vi "Heapify.vi"(8 "error in (no error)":errorcluster, 10 "index":i32, 11 "Astar Open List in":refnum<class "NI_Robotics_Priority Queue.lvclass">) -> (0 "error out":errorcluster, 3 "Astar Open List out":refnum<class "NI_Robotics_Priority Queue.lvclass">)   [LabVIEW 2017, in "NI_Robotics_Priority Queue.lvclass"]
uses:
  <vilib>/robotics/Navigation/shared/Priority Queue/NI_Robotics_Priority Queue.lvclass
panel:
  in  "up heap (F)":bool
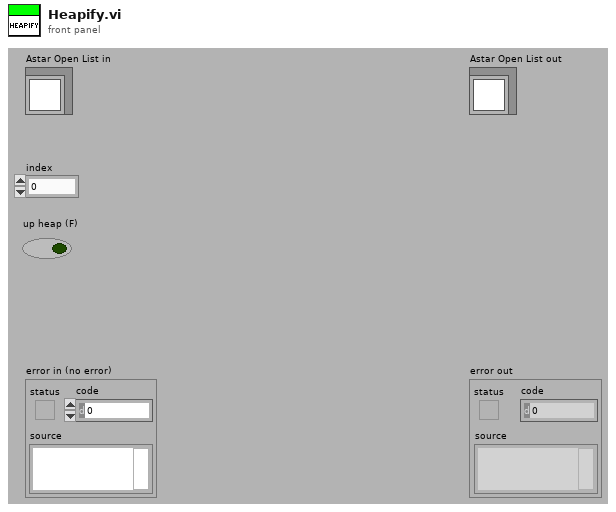
[diagram p1: front panel]
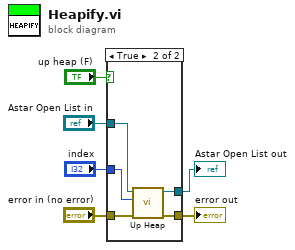
[diagram p0: block diagram]
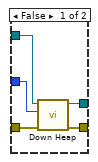
[diagram p2: hidden frame]
diagram:
  n1 = case shown="True" "up heap (F)" {
    tunnel: "Astar Open List in" -> [w11 w16]
    tunnel: "index" -> [w10 w15]
    tunnel: [w9 w13] -> w3
    tunnel: "error in (no error)" -> [w8 w14]
    tunnel: [w7 w12] -> w1
    frame False {
      n2 = call <vilib>:"Down Heap.vi"("error in (no error)"=w8, "index"=w10, "Astar Open List in"=w11) -> ("error out"=w7:errorcluster, "Astar Open List out"=w9:refnum<class "NI_Robotics_Priority Queue.lvclass">)  [unwired: 7 in]
    }
    frame True {
      n3 = call <vilib>:"Up Heap.vi"("error in (no error)"=w14, "index"=w15, "Astar Open List in"=w16) -> ("error out"=w12:errorcluster, "Astar Open List out"=w13:refnum<class "NI_Robotics_Priority Queue.lvclass">)  [unwired: 7 in]
    }
  }
  "error out" <- w1
  "Astar Open List out" <- w3
